vi "PassThru.vi"(8 "error in (no error)":errorcluster, 9 "timeout ms (1000)":i32=1000, 10 "Frame":T1 {"payload" format="%x"; "timestamp" format="%<%.7X\n%x>T"; "type" items=["CAN Data"=0, "CAN Remote"=1, "CAN Bus Error"=2, "CAN 2.0 Data"=8, "CAN FD Data"=16, "CAN FD+BRS Data"=24, "J1939 Data"=192, "Delay"=224, "Log Trigger"=225, "Start Trigger"=226]; "identifier" format="%x"}, 11 "Ref in":T3) -> (0 "error out":errorcluster, 3 "Ref out":T3)   [LabVIEW 2019, in "Protection and Counter Host Automation API.lvlib"]
uses:
  Protection and Counter Host Automation API.lvlib
  Types/API Variables.ctl
  <vilib>/NI/STM/TCP/TCP Connection Info.ctl
  <vilib>/NI/STM/SubVIs/MetaDataElement.ctl
  <vilib>/xnet/xnet.llb/XNET Frame CAN.ctl
  <vilib>/xnet/xnet.llb/XNET Frame Type CAN.ctl
  <vilib>/NI/NI VeriStand Addon Network Comm/Shared/NI VeriStand Addon Network Comm Shared.lvlib
  <vilib>/NI/STM/NI STM.lvlib
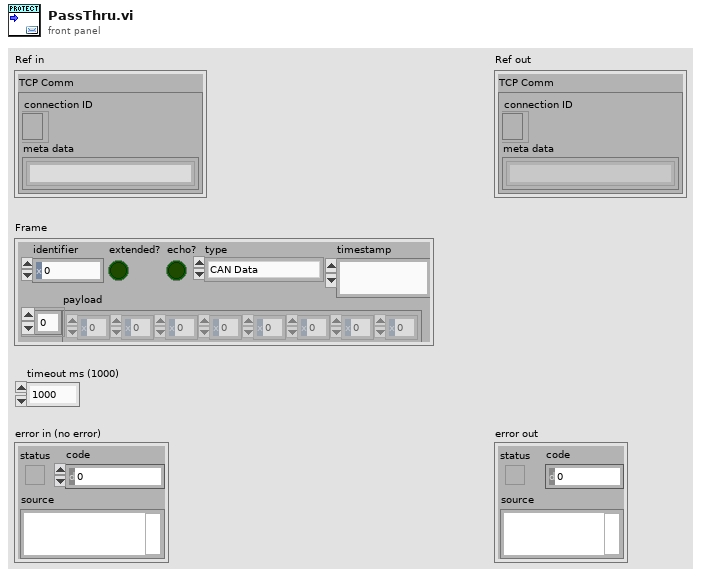
[diagram p1: front panel]
types:
  T1 = typedef "XNET Frame CAN.ctl" = cluster{"timestamp":timestamp, "payload":u8[], "identifier":u32, "type":T2, "extended?":bool, "echo?":bool}
  T2 = typedef "XNET Frame Type CAN.ctl" = u8
  T3 = typedef "Protection and Counter Host Automation API.lvlib/API Variables.ctl" = cluster{"TCP Comm":T4}
  T4 = typedef "NI STM.lvlib/TCP Connection Info.ctl" = cluster{"connection ID":refnum<k5>, "meta data":T5[]}
  T5 = typedef "NI STM.lvlib/MetaDataElement.ctl" = string
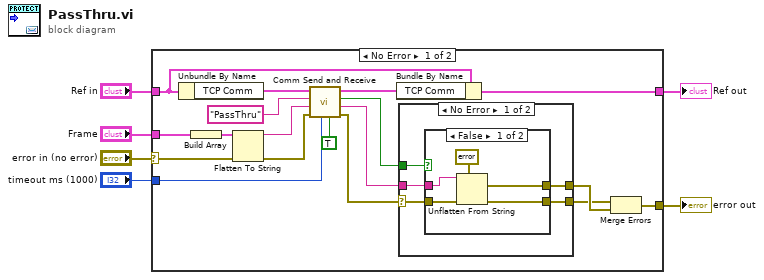
[diagram p0: block diagram]
diagram:
  n1 = case shown="No Error" "error in (no error)" {
    selector: "error in (no error)" -> [w24 w38]
    tunnel: "Ref in" -> [w13 w37]
    tunnel: [w11 w37] -> w3
    tunnel: [w8 w38] -> w2
    tunnel: "timeout ms (1000)" -> [w15 _]
    tunnel: "Frame" -> [w23 _]
    frame No Error {
      n2 = Unbundle By Name(w13) -> ("TCP Comm"=w14:T4)
      n3 = Build Array(w23) -> (w7:T1[])
      n4 = Flatten To String(anything=w7, error in (no error)=w24) -> (data string=w17:string, error out=w18:errorcluster)  [unwired: 2 in, 1 out]
      n5 = call <vilib>:"Comm Send and Receive.vi"("Resp Required?"=TRUE, "Timeout (ms)"=w15, "error in (no error)"=w18, "Data"=w17, "Name"="PassThru", "connection info"=w14) -> ("error out"=w19:errorcluster, "Data"=w20:string, "Timed Out?"=w21:bool, "connection info"=w12:T4)  [unwired: 2 in]
      n6 = Bundle By Name(cluster=w13, "TCP Comm"=w12) -> (w11:T3)
      n7 = case shown="No Error" w19 {
        selector: w19 -> [w27 w36]
        tunnel: w21 -> [w29 _]
        tunnel: [w28 w36] -> w9
        tunnel: w20 -> [w26 _]
        tunnel: [w25 _] -> w10
        frame No Error {
          n8 = case shown="False" w29 {
            tunnel: [w32 w35] -> w28
            tunnel: w27 -> [w33 w35]
            tunnel: w26 -> [w34 _]
            tunnel: [w31 _] -> w25
            frame False {
              n9 = Unflatten From String(type=errorcluster {"status"=FALSE, "code"=0, "source"=""} ("error IO"), binary string=w34, error in (no error)=w33) -> (value=w31:errorcluster, error out=w32:errorcluster)  [unwired: 2 in, 1 out]
            }
            frame True {
            }
          }
        }
        frame Error {
        }
      }
      n10 = Merge Errors(w9, w10) -> (w8:errorcluster)
    }
    frame Error {
    }
  }
  "error out" <- w2
  "Ref out" <- w3
